vi "Minute.vi"(8 "error in (no error)":errorcluster, 11 "Blueprint in":refnum<class "Blueprint.lvclass">) -> (0 "error out":errorcluster, 3 "Blueprint out":refnum<class "Blueprint.lvclass">)   [LabVIEW 2021, in "d19.lvlib" / "Blueprint.lvclass"]
uses:
  Blueprint.lvclass
  Blueprint.lvclass/Blueprint.ctl
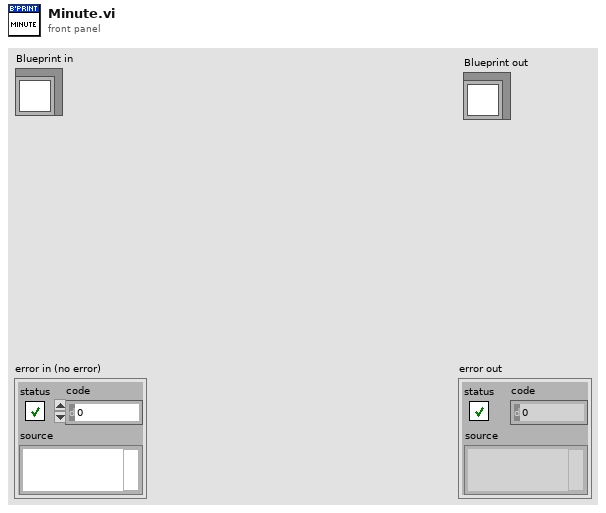
[diagram p1: front panel]
types:
  T1 = cluster{"Robots[0]":u64, "Robots[1]":u64, "Robots[2]":u64, "Robots[3]":u64}
  T2 = cluster{"Ore":i64, "Clay":i64, "Obsidian":i64, "Geodes":i64}
  T3 = cluster{"Ore":u64, "Clay":u64, "Obsidian":u64, "Geodes":u64}
  T4 = cluster{"Ore":cluster{"Ore":u64, "Clay":u64, "Obsidian":u64, "Geodes":u64}, "Clay":cluster{"Ore":u64, "Clay":u64, "Obsidian":u64, "Geodes":u64}, "Obsidian":cluster{"Ore":u64, "Clay":u64, "Obsidian":u64, "Geodes":u64}, "Geode":cluster{"Ore":u64, "Clay":u64, "Obsidian":u64, "Geodes":u64}}
  T5 = cluster{"Ore":u64, "Clay":u64, "Obsidian":u64, "Geodes":u64}[]
  T6 = cluster{"[0]":u64, "[1]":u64, "[2]":u64, "[3]":u64}
  T7 = cluster{"f[0]":u64, "f[1]":u64, "f[2]":u64, "f[3]":u64}
  T8 = cluster{"Ore":bool, "Clay":bool, "Obsidian":bool, "Geodes":bool}
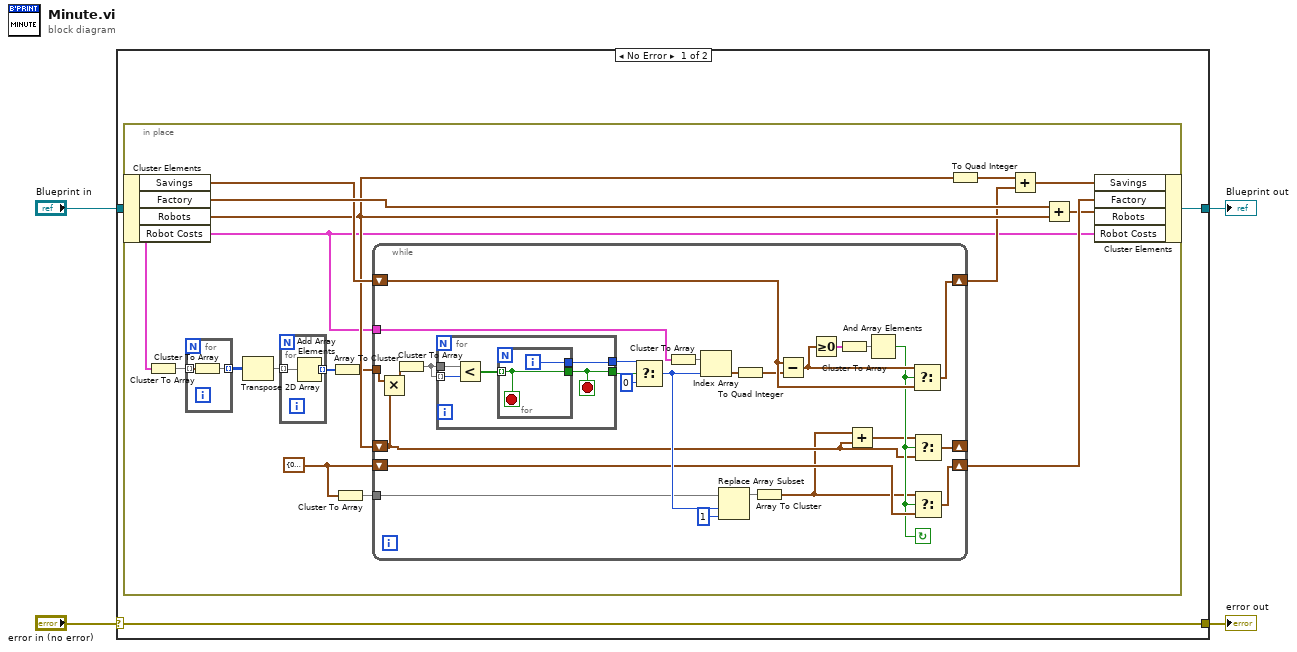
[diagram p0: block diagram]
diagram:
  n1 = case shown="No Error" "error in (no error)" {
    selector: "error in (no error)" -> [w7 w62]
    tunnel: [w7 w62] -> w3
    tunnel: [w5 w61] -> w1
    tunnel: "Blueprint in" -> [w6 w61]
    frame No Error {
      n2 = in-place {
        w16 = T1 {"Robots[0]"=0, "Robots[1]"=0, "Robots[2]"=0, "Robots[3]"=0} ("f")
        n3 = in-place-cluster #1(w6) -> ("Savings"=w20:T2, "Factory"=w23:T3, "Robots"=w18:T3, "Robot Costs"=w13:T4)
        n4 = Cluster To Array(cluster=w13) -> (array=w12:T5)
        n5 = for {
          tunnel: w12 -> [w27] mode=indexing
          tunnel: [w26] -> w11 mode=indexing
          n6 = Cluster To Array(cluster=w27) -> (array=w26:u64[])
        }
        n7 = Transpose 2D Array(2D array=w11) -> (transposed array=w10:u64[][])
        n8 = for {
          tunnel: w10 -> [w25] mode=indexing
          tunnel: [w24] -> w9 mode=indexing
          n9 = Add Array Elements(numeric array=w25) -> (sum=w24:u64)
        }
        n10 = Array To Cluster(array=w9) -> (cluster=w8:T6)
        n11 = Cluster To Array(cluster=w16) -> (array=w15:u64[])
        n12 = while {
          tunnel: w13 -> [w53]
          shift-right: [w45] -> w14
          shift-left: w20 -> [w40]
          shift-right: [w34] -> _
          shift-left: w18 -> [w32]
          shift-right: [w41] -> w22
          shift-left: w16 -> [w37]
          tunnel: w15 -> [w36]
          tunnel: w8 -> [w28]
          stop <- w33 continue-if-true
          n13 = Multiply(x=w28, y=w32) -> (x*y=w29:cluster{u64, u64, u64, u64})
          n14 = Cluster To Array(cluster=w29) -> (array=w43:u64[])
          n15 = for {
            tunnel: w43 -> [w58] mode=indexing
            tunnel: w43 -> [w56]
            tunnel: [w55] -> w51
            tunnel: [w54] -> w52
            stop <- w54 stop-if-true
            n16 = Less?(x=w56, y=w58) -> (x < y?=w57:bool[])
            n17 = for {
              tunnel: w57 -> [w59] mode=indexing
              tunnel: [w60] -> w55
              tunnel: [w59] -> w54
              i -> [w60]
              stop <- w59 stop-if-true
            }
          }
          n18 = Select(t=w51, s=w52, f=0) -> (s? t:f=w44:i32)
          n19 = Cluster To Array(cluster=w53) -> (array=w49:T5)
          n20 = Index Array(array=w49, index=w44) -> (element=w46:T3)
          n21 = Replace Array Subset(array=w36, new element=u64 1 ("new element/subarray"), index=w44) -> (w42:u64[])
          n22 = To Quad Integer(1:w46) -> (0:w39:T2)
          n23 = Array To Cluster(array=w42) -> (cluster=w31:T7)
          n24 = Subtract(x=w40, y=w39) -> (x-y=w38:T2)
          n25 = Greater Or Equal To 0?(x=w38) -> (x >= 0?=w48:T8)
          n26 = Cluster To Array(cluster=w48) -> (array=w47:bool[])
          n27 = Add(x=w31, y=w32) -> (x+y=w30:cluster{u64, u64, u64, u64})
          n28 = And Array Elements(Boolean array=w47) -> (logical AND=w33:bool)
          n29 = Select(t=w38, s=w33, f=w40) -> (s? t:f=w45:T2)
          n30 = Select(t=w30, s=w33, f=w32) -> (s? t:f=w34:T3)
          n31 = Select(t=w31, s=w33, f=w37) -> (s? t:f=w41:T1)
        }
        n32 = To Quad Integer(1:w18) -> (0:w17:T2)
        n33 = Add(x=w17, y=w14) -> (x+y=w19:T2)
        n34 = Add(x=w23, y=w18) -> (x+y=w21:T3)
        n35 = in-place-cluster #1("Savings"=w19, "Factory"=w22, "Robots"=w21, "Robot Costs"=w13) -> (w5:refnum<class "Blueprint.lvclass">)
      }
    }
    frame Error {
    }
  }
  "error out" <- w3
  "Blueprint out" <- w1
